vi "PrepareData4HTML.vi"(6 "Root":path, 9 "Glyphs []":T1[](array[typedef]), 11 "Header":string) -> (1 "HTML String":string)   [LabVIEW 2020]
uses:
  vi.lib/LabVIEW Icon API/lv_icon/Controls/Graphic.ctl
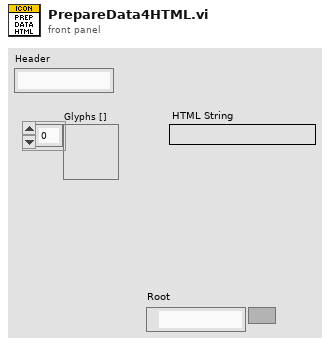
[diagram p1: front panel]
types:
  T1 = typedef "Graphic.ctl" = cluster{"Rectangle":cluster{"left":i16, "top":i16, "right":i16, "bottom":i16}, "Path":path, "Image":picture, "Filter":string, "FileName":string}
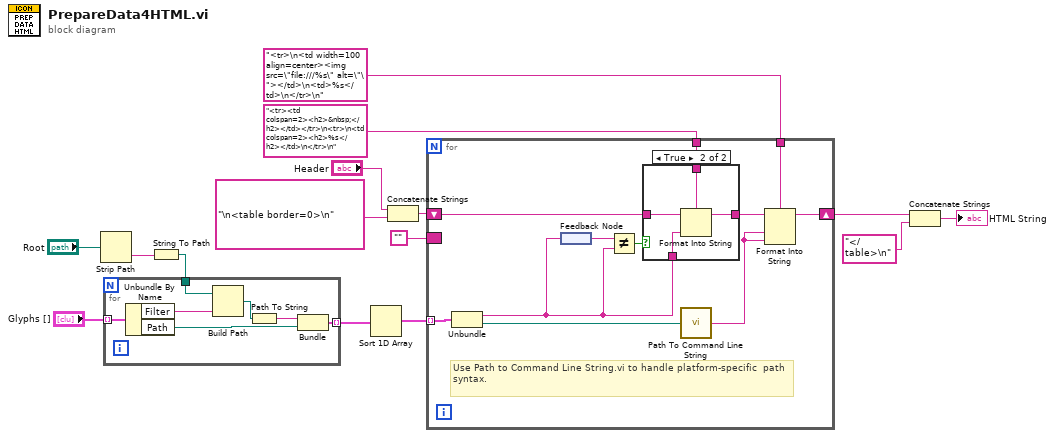
[diagram p0: block diagram]
diagram:
  n1 = Strip Path(path="Root") -> (name=w2:string)  [unwired: 1 out]
  n2 = String To Path(string=w2) -> (path=w1:path)
  n3 = for {
    tunnel: "Glyphs []" -> [w22] mode=indexing
    tunnel: [w20] -> w12 mode=indexing
    tunnel: w1 -> [w17]
    n4 = Unbundle By Name(w22) -> ("Filter"=w16:string, "Path"=w21:path)
    n5 = Build Path(base path=w17, name or relative path=w16) -> (appended path=w19:path)
    n6 = Path To String(path=w19) -> (string=w18:string)
    n7 = Bundle(w18, "Path"=w21) -> (w20:cluster{string, "Path":path})  [unwired: 1 out]
  }
  n8 = Sort 1D Array(array=w12) -> (sorted array=w13:cluster{string, "Path":path}[])
  n9 = Concatenate Strings("Header", "\n<table border=0>\n") -> (w4:string)
  n10 = for {
    tunnel: w13 -> [w33] mode=indexing
    shift-right: [w26] -> w9
    shift-left: w4 -> [w31]
    tunnel: "<tr><td colspan=2><h2>&nbsp;</h2></td></tr>\n<tr>\n<td colspan=2><h2>%s</h2></td>\n</tr>\n" -> [w30]
    tunnel: "<tr>\n<td width=100 align=center><img src=\"file:///%s\" alt=\"\"></td>\n<td>%s</td>\n</tr>\n" -> [w28]
    border: "" -> [_]
    # "Use Path to Command Line String.vi to handle platform-specific  path syntax."
    n11 = Unbundle(w33) -> (w25:string, "Path"=w27:path)
    n12 = feedback-in #1(w25) -> ()
    n13 = feedback #1() -> (w24:string)
    n14 = Not Equal?(x=w24, y=w25) -> (x != y?=w32:bool)
    n15 = case shown="True" w32 {
      tunnel: w31 -> [w34 w37]
      tunnel: w30 -> [_ w38]
      tunnel: w25 -> [_ w36]
      tunnel: [w34 w35] -> w29
      frame False {
      }
      frame True {
        n16 = Format Into String(format string=w38, initial string=w37, w36) -> (resulting string=w35:string)  [unwired: 1 in, 1 out]
      }
    }
    n17 = call <vilib>:"Path To Command Line String.vi"("path"=w27) -> ("string"=w23:string)
    n18 = Format Into String(format string=w28, initial string=w29, w23, w23) -> (resulting string=w26:string)  [unwired: 1 in, 1 out]
  }
  n19 = Concatenate Strings(w9, "</table>\n" ("string")) -> (→"HTML String":string)
